vi "Save.vi"(8 "error in (no error)":errorcluster, 9 "Overlays (None)":refnum<class "Config Storage.lvclass">[](array[class]), 10 "Config":refnum<class "Config Manager.lvclass">, 11 "Config Storage in":refnum<class "Config Storage.lvclass">) -> (0 "error out":errorcluster, 3 "Config Storage out":refnum<class "Config Storage.lvclass">)   [LabVIEW 2020, in "CDM-Config.lvlib" / "Config Storage.lvclass"]
doc: "Persists the configuration tree to the child implemented format from the specified config instance. This optionally accepts <b>Overlays</b> which saves the same configs with additional filters defined. This is useful for saving parts of a config as a separate file, such as specific meta data fields or specific subtrees."
uses:
  Config Storage.lvclass
  Config Manager/Config Manager.lvclass
  Config Storage.lvclass/Config Storage.ctl
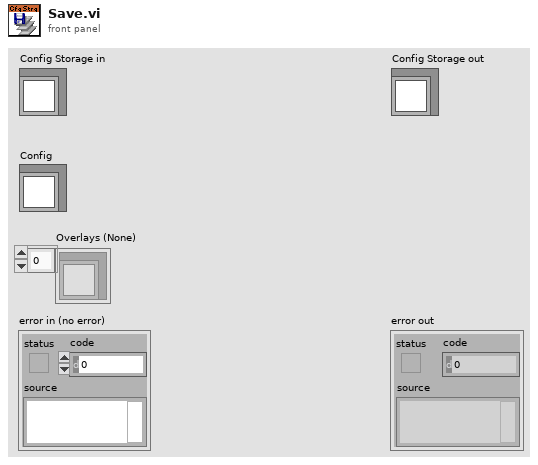
[diagram p1: front panel]
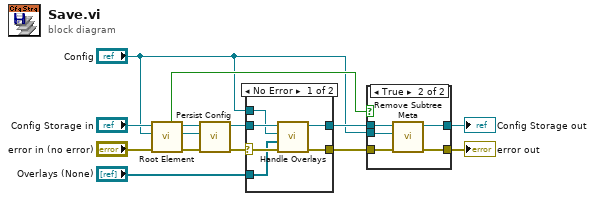
[diagram p0: block diagram]
diagram:
  n1 = call "Root Element.vi"("error in (no error)"="error in (no error)", "Config"="Config", "Config Storage in"="Config Storage in") -> ("error out"=w10:errorcluster, "Root"=w7:refnum<class "Config Element.lvclass">, "Config Storage out"=w8:refnum<class "Config Storage.lvclass">, "Subtree Added"=w5:bool)  [unwired: 5 in]
  n2 = call-dynamic "Persist Config.vi"("error in (no error)"=w10, "Root"=w7, "Config Storage in"=w8) -> ("error out"=w13:errorcluster, "Config Storage out"=w12:refnum<class "Config Storage.lvclass">)  [unwired: 7 in]
  n3 = case shown="No Error" w13 {
    selector: w13 -> [w19 w21]
    tunnel: w12 -> [w20 w22]
    tunnel: "Config" -> [w18 _]
    tunnel: [w17 w21] -> w6
    tunnel: [w16 w22] -> w4
    tunnel: "Overlays (None)" -> [w15 _]
    frame No Error {
      n4 = call "Handle Overlays.vi"("error in (no error)"=w19, "Overlays"=w15, "Config"=w18, "Config Storage in"=w20) -> ("error out"=w17:errorcluster, "Config Storage out"=w16:refnum<class "Config Storage.lvclass">)  [unwired: 6 in]
    }
    frame Error {
    }
  }
  n5 = case shown="True" w5 {
    tunnel: w6 -> [w23 w28]
    tunnel: w4 -> [w24 w29]
    tunnel: "Config" -> [_ w27]
    tunnel: [w24 w26] -> w2
    tunnel: [w23 w25] -> w1
    frame False {
    }
    frame True {
      n6 = call "Remove Subtree Meta.vi"("error in (no error)"=w28, "Config"=w27, "Config Storage in"=w29) -> ("error out"=w25:errorcluster, "Config Storage out"=w26:refnum<class "Config Storage.lvclass">)  [unwired: 7 in]
    }
  }
  "error out" <- w1
  "Config Storage out" <- w2
